vi "marshalling.vi"(8 "error in (no error)":errorcluster, 10 "Variant":variant, 11 "CustomFlat in":refnum<class "CustomFlat.lvclass">) -> (0 "error out":errorcluster, 2 "String":string, 3 "CustomFlat out":refnum<class "CustomFlat.lvclass">)   [LabVIEW 2023, in "CustomFlat.lvclass"]
uses:
  CustomFlat.lvclass
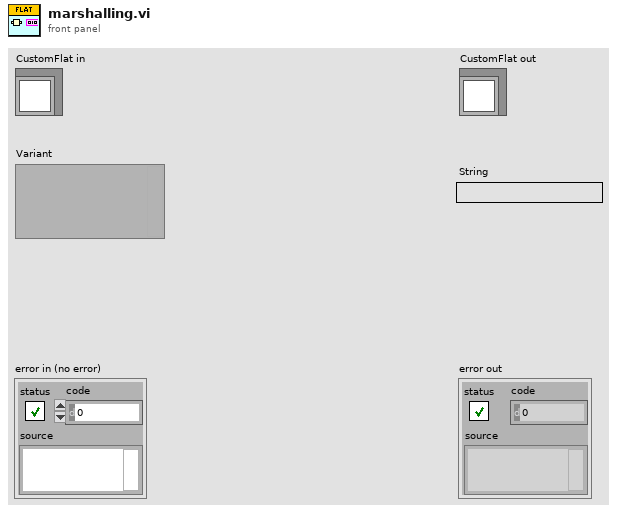
[diagram p1: front panel]
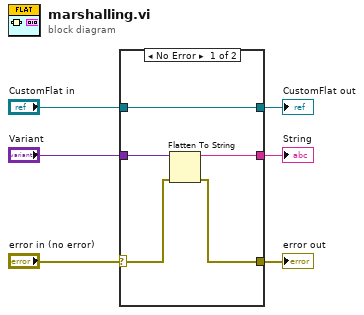
[diagram p0: block diagram]
diagram:
  n1 = case shown="No Error" "error in (no error)" {
    selector: "error in (no error)" -> [w8 w12]
    tunnel: "Variant" -> [w10 _]
    tunnel: "CustomFlat in" -> [w11 w13]
    tunnel: [w11 w13] -> w3
    tunnel: [w9 _] -> w2
    tunnel: [w7 w12] -> w1
    frame No Error {
      n2 = Flatten To String(anything=w10, error in (no error)=w8) -> (data string=w9:string, error out=w7:errorcluster)  [unwired: 2 in, 1 out]
    }
    frame Error {
    }
  }
  "error out" <- w1
  "CustomFlat out" <- w3
  "String" <- w2
